vi "Timing_AnalogOut.vi"() -> ()   [LabVIEW 2016]
uses:
  <vilib>/Platform/TimedLoop/XDataNode/timing_clust.ctl
  <vilib>/Platform/TimedLoop/XDataNode/nitl_modes.ctl
  <vilib>/Platform/TimedLoop/XDataNode/wakeup.ctl
  <vilib>/rvi/Emulation/niFpgaGetClockAttributes.vi
  <vilib>/rvi/Emulation/niFpgaSctlEmulationGetInTimedLoop.vi
  <vilib>/rvi/Emulation/niFpgaEmulationReportErrorSimple.vi
  <vilib>/rvi/Emulation/niFpgaCriticalErrorInLSC.vi
  <vilib>/rvi/eio/common/nirviEmuTemplateMethod_errors.vi
  <vilib>/Platform/TimedLoop/XDataNode/XDataNode.xnode
  <vilib>/eio/EIONode/EIONode.xnode
  <vilib>/Platform/TimedLoop/XDataNode/XDNodeRunTimeDep.lvlib
panel:
  out "Ticks":u32
  in  "stop":bool
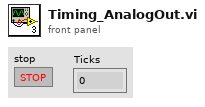
[diagram p1: front panel]
types:
  T1 = typedef "XDNodeRunTimeDep.lvlib/timing_clust.ctl" = cluster{"Expected End [f-1]":u64, "Actual End [f-1]":u64, "Finished Late? [f-1]":bool, "Expected End [i-1]":u64, "Actual End [i-1]":u64, "Finished Late? [i-1]":bool, "Expected Start [i]":u64, "Actual Start [i]":u64, "Expected Start [f]":u64, "Actual Start [f]":u64, "Source Name":string, "Structure Name":string, "Period":i64, "Deadline":i64, "Offset":i64, "Start":i64, "Priority":i32, "Timeout":i32, "Mode":T2, "Wakeup Reason":T3, "Error":errorcluster, "Source Type":string, "Secondary Source Type":string, "Global End Time":u64, "Global Start Time":u64, "Frame Duration":u64, "Iteration Duration":u64, "Assigned CPU":i32, "I/O Scan Engine Mode":u32}
  T2 = typedef "XDNodeRunTimeDep.lvlib/nitl_modes.ctl" = enum32{"No Change", "Process missed periods, maintain original phase", "Discard missed periods, maintain original phase", "Process missed periods, ignore original phase", "Discard missed periods, ignore original phase"}
  T3 = typedef "XDNodeRunTimeDep.lvlib/wakeup.ctl" = enum32{"Normal", "Aborted", "Asynchronous wakeup", "Timing source error", "Timed loop error", "Timeout"}
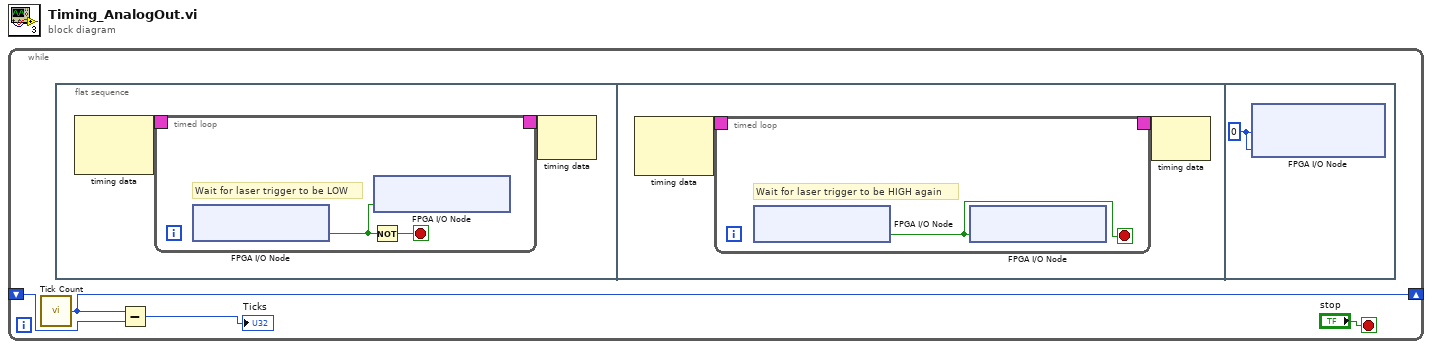
[diagram p0: block diagram]
diagram:
  n1 = while {
    shift-right: [w2] -> _
    shift-left: _ -> [w3]
    stop <- "stop" stop-if-true
    n2 = call "Tick Count"() -> ("Tick Count(Ticks)"=w2:u32)
    n3 = flat-sequence {
      frame #0 {
        n4 = node-c288() -> (w6:T1)  [unwired: 2 in]
        n5 = timed-loop {
          timing: w6 -> [_]
          timing-out: [_] -> w5
          stop <- w7 stop-if-true
          # "Wait for laser trigger to be LOW"
          n6 = xnode "FPGA I/O Node"() -> ("Connector0/DIO4"=w8:bool)  [unwired: 1 in, 1 out]
          n7 = Not(x=w8) -> (.not. x?=w7:bool)
          n8 = xnode "FPGA I/O Node"("Connector0/DIO0"=w8) -> ()  [unwired: 1 in, 1 out]
        }
        n9 = node-c288(w5) -> ()  [unwired: 1 out]
      }
      frame #1 {
        n10 = node-c288() -> (w14:T1)  [unwired: 2 in]
        n11 = timed-loop {
          timing: w14 -> [_]
          timing-out: [_] -> w13
          stop <- w15 stop-if-true
          # "Wait for laser trigger to be HIGH again"
          n12 = xnode "FPGA I/O Node"() -> ("Connector0/DIO4"=w15:bool)  [unwired: 1 in, 1 out]
          n13 = xnode "FPGA I/O Node"("Connector0/DIO0"=w15) -> ()  [unwired: 1 in, 1 out]
        }
        n14 = node-c288(w13) -> ()  [unwired: 1 out]
      }
      frame #2 {
        w20 = i16 0 ("Connector0/AO0")
        n15 = xnode "FPGA I/O Node"("Connector0/AO0"=w20, "Connector0/AO1"=w20) -> ()  [unwired: 2 in, 2 out]
      }
    }
    n16 = Subtract(x=w2, y=w3) -> (x-y=→"Ticks":u32)
  }
